vi "Preview Dialog.vi"(8 "error in":errorcluster, 10 "current configuration":T1, 11 "new configuration":T1) -> (0 "error out":errorcluster, 3 "apply changes":bool)   [LabVIEW 2020, in "AIM MIL-STD-1553 System Explorer.lvlib" / "Implementation.lvlib" / "Refresh.lvlib"]
uses:
  Refresh.lvlib
  <vilib>/Utility/miscctls.llb/LVRowAndColumnUnsignedTypeDef.ctl
  <vilib>/Utility/miscctls.llb/LVRowAndColumnTypeDef.ctl
  Shared/Address.ctl
  Shared/Terminal Endpoint.ctl
  Shared/Parameter Definition.ctl
  Shared/Message Type.ctl
  Shared/Message Definition.ctl
  Shared/BIU Configuration.ctl
  Shared/Major Frame Definition.ctl
  Shared/Minor Frame Definition.ctl
  Shared/Acyclic Frame Definition.ctl
panel:
  out "changes preview":i32(listbox)
  in  "changes only":bool=TRUE
  in  "Cancel":bool
  in  "OK":bool
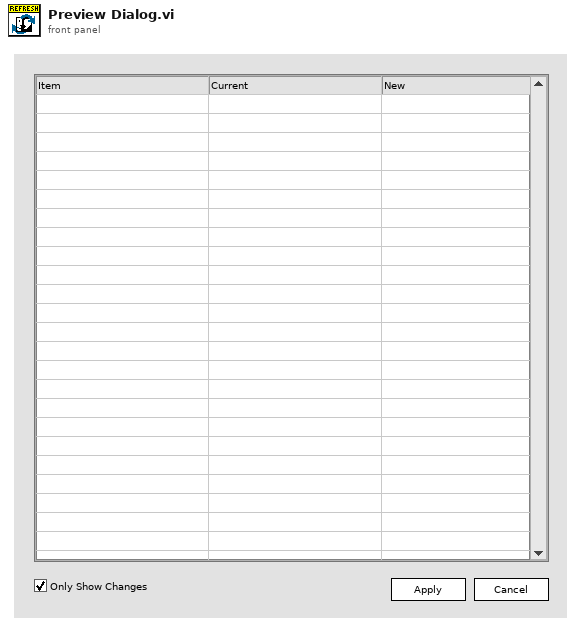
[diagram p1: front panel]
types:
  T1 = typedef "BIU Configuration.ctl" = cluster{"HW channel":u16, "terminal addresses":T2[], "terminal names":string[], "major frames":T3[], "minor frames":T4[], "acyclic frames":T5[], "messages":T6[]}
  T2 = typedef "Address.ctl" = u16
  T3 = typedef "Major Frame Definition.ctl" = cluster{"name":string, "minor frames":string[]}
  T4 = typedef "Minor Frame Definition.ctl" = cluster{"name":string, "messages":string[]}
  T5 = typedef "Acyclic Frame Definition.ctl" = cluster{"name":string, "messages":string[]}
  T6 = typedef "Message Definition.ctl" = cluster{"name":string, "message type":T7, "endpoint Tx":T8, "endpoint Rx":T8, "create timestamp channel":bool, "mode code":u16, "number of words":u16, "parameters":cluster{"name":string, "default value":dbl, "unit":string, "parameter definition":T9}[]}
  T7 = typedef "Message Type.ctl" = string
  T8 = typedef "Terminal Endpoint.ctl" = cluster{"terminal address":T2, "subaddress":T2}
  T9 = typedef "Parameter Definition.ctl" = cluster{"start index":i32, "size (bits)":i32, "encoding":enum16{"BNR", "BCD", "Discrete"}, "signed":bool, "multiplier":dbl, "offset":dbl}
  T10 = typedef "AIM MIL-STD-1553 System Explorer.lvlib/Implementation.lvlib/Refresh.lvlib/MCL Row.ctl" = cluster{"change type":T11, "item symbol":T12, "item names":string[]}
  T11 = typedef "AIM MIL-STD-1553 System Explorer.lvlib/Implementation.lvlib/Refresh.lvlib/Change Type.ctl" = enum16{"No change", "Modify", "Add", "Remove"}
  T12 = typedef "AIM MIL-STD-1553 System Explorer.lvlib/Implementation.lvlib/Refresh.lvlib/Symbols.ctl" = enum16{"Blank", "MIL-STD-1553", "Port", "Remote Terminal", "Subaddress", "Bus Controller", "Acyclic Frame", "Mode Code", "Message", "Parameter", "Item"}
  T13 = typedef "imagedata.ctl" = cluster{"image type":i32, "image depth":i32, "image":u8[], "mask":u8[], "colors":u32[], "Rectangle":cluster{"left":i16, "top":i16, "right":i16, "bottom":i16}}
  T14 = typedef "LVRowAndColumnUnsignedTypeDef.ctl" = cluster{"Row":u32, "Column":u32}
  T15 = typedef "LVRowAndColumnTypeDef.ctl" = cluster{"Row":i32, "Column":i32}
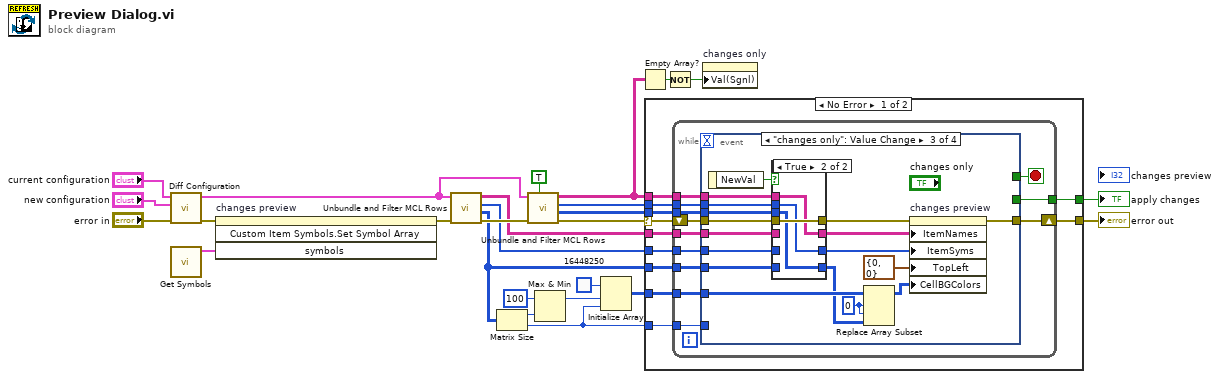
[diagram p0: block diagram]
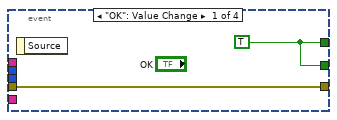
[diagram p2: hidden frame]
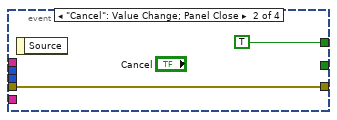
[diagram p3: hidden frame]
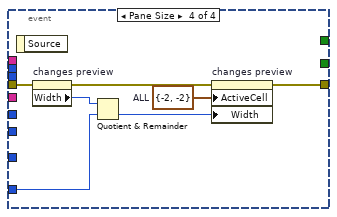
[diagram p5: hidden frame]
diagram:
  n1 = call "Diff Configuration.vi"("error in"="error in", "configuration new"="new configuration", "configuration old"="current configuration") -> ("error out"=w25:errorcluster, "configuration diff"=w20:T10[])  [unwired: 7 in]
  n2 = call "Get Symbols.vi"() -> ("MIL-STD-1553 symbols"=w26:T13[])  [unwired: 11 in]
  n3 = invoke on="changes preview" class="MCListbox (strict)" method="Custom Item Symbols.Set Symbol Array"(error in=w25, "symbols"=w26) -> (error out=w5:errorcluster)  [unwired: 2 in, 3 out]
  n4 = call "Unbundle and Filter MCL Rows.vi"("error in"=w5, "refresh items"=w20) -> ("error out"=w22:errorcluster, "background colors"=w1:u32[][], "item symbols"=w15:T12[], "item names"=w16:string[][])  [unwired: 6 in]
  n5 = Matrix Size(0:w1) -> (1:w10:i32, 2:w9:i32)
  n6 = call "Unbundle and Filter MCL Rows.vi"("filter changed items"=TRUE, "error in"=w22, "refresh items"=w20) -> ("error out"=w21:errorcluster, "background colors"=w17:u32[][], "item symbols"=w18:T12[], "item names"=w4:string[][])  [unwired: 5 in]
  n7 = Max & Min(x=100 ("maximum expected visible rows"), y=w10) -> (max(x,y)=w11:i32)  [unwired: 1 out]
  n8 = Initialize Array(u32 16448250, w11, w9) -> (w13:u32[][])
  n9 = Empty Array?(array=w4) -> (empty?=w3:bool)
  n10 = case shown="No Error" w21 {
    selector: w21 -> [w36 w86]
    tunnel: [w35 w86] -> w24
    tunnel: [w37 _] -> w23
    tunnel: w4 -> [w34 _]
    tunnel: w18 -> [w33 _]
    tunnel: w17 -> [w32 _]
    tunnel: w16 -> [w31 _]
    tunnel: w15 -> [w30 _]
    tunnel: w1 -> [w29 _]
    tunnel: w13 -> [w28 _]
    tunnel: w9 -> [w27 _]
    frame No Error {
      n11 = while {
        tunnel: [w49] -> w37
        shift-right: [w46] -> w35
        shift-left: w36 -> [w47]
        tunnel: w34 -> [w45]
        tunnel: w33 -> [w44]
        tunnel: w32 -> [w43]
        tunnel: w31 -> [w42]
        tunnel: w30 -> [w41]
        tunnel: w29 -> [w40]
        tunnel: w28 -> [w39]
        tunnel: w27 -> [w38]
        stop <- w48 stop-if-true
        n12 = event shown="[2] \"changes only\": Value Change" {
          selector: _ -> [_ _ _ _]
          dyn-events: _ -> [_ _ _ _]
          timeout: _ -> [_ _ _ _]
          tunnel: [w51 _ _ _] -> w49
          tunnel: [w51 TRUE ("OK") _ _] -> w48
          tunnel: w47 -> [w50 w52 w60 w85]
          tunnel: [w50 w52 w70 w79] -> w46
          tunnel: w45 -> [_ _ w64 _]
          tunnel: w44 -> [_ _ w63 _]
          tunnel: w43 -> [_ _ w62 _]
          tunnel: w42 -> [_ _ w68 _]
          tunnel: w41 -> [_ _ w66 _]
          tunnel: w40 -> [_ _ w65 _]
          tunnel: w39 -> [_ _ w57 _]
          tunnel: w38 -> [_ _ _ w82]
          event "OK": Value Change {
            w51 = TRUE ("OK")
            n13 = event-data() -> ()  [unwired: 1 in, 1 out]
          }
          event "Cancel": Value Change; Panel Close {
            n14 = event-data() -> ()  [unwired: 1 in, 1 out]
          }
          event "changes only": Value Change {
            w58 = 0 ("index (row)")
            n15 = event-data() -> ("NewVal"=w59:bool)  [unwired: 1 in]
            n16 = case shown="True" w59 {
              tunnel: [w74 w77] -> w69
              tunnel: w68 -> [w74 _]
              tunnel: [w73 w76] -> w67
              tunnel: w66 -> [w73 _]
              tunnel: [w72 w75] -> w56
              tunnel: w65 -> [w72 _]
              tunnel: w64 -> [_ w77]
              tunnel: w63 -> [_ w76]
              tunnel: w62 -> [_ w75]
              tunnel: [w71 w78] -> w61
              tunnel: w60 -> [w71 w78]
              frame False {
              }
              frame True {
              }
            }
            n17 = Replace Array Subset(array=w57, new element=w56, index (row)=w58, index (col)=w58) -> (w55:u32[][])
            n18 = property on="changes preview" class="MCListbox (strict)"(error in=w61, "ItemNames"=w69, "ItemSyms"=w67, "TopLeft"=T14 {"Row"=0, "Column"=0} ("Top Left Visible Cell"), "CellBGColors"=w55) -> (error out=w70:errorcluster)  [unwired: 1 in, 1 out]
          }
          event Pane Size {
            w84 = T15 {"Row"=-2, "Column"=-2}  # ALL
            n19 = event-data() -> ()  [unwired: 1 in, 1 out]
            n20 = property on="changes preview" class="MCListbox (strict)"(error in=w85) -> (error out=w80:errorcluster, "Width"=w83:u32)  [unwired: 1 in, 1 out]
            n21 = Quotient & Remainder(x=w83, y=w82) -> (floor(x/y)=w81:u32)  [unwired: 1 out]
            n22 = property on="changes preview" class="MCListbox (strict)"(error in=w80, "ActiveCell"=w84, "Width"=w81) -> (error out=w79:errorcluster)  [unwired: 1 in, 1 out]
          }
        }
      }
    }
    frame Error {
    }
  }
  "error out" <- w24
  "apply changes" <- w23
  n23 = Not(x=w3) -> (.not. x?=w2:bool)
  n24 = property on="changes only" class="Bool (strict)"("Val(Sgnl)"=w2) -> ()  [unwired: 2 in, 2 out]
